vi "GlobalVariables.vi"() -> ()   [LabVIEW 2014]
panel:
  out "FPGA VI Reference Out":refnum<k20>
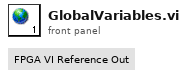
[diagram p1: front panel]
diagram:
